vi "P3.6.vi"() -> ()   [LabVIEW 2020]
uses:
  <vilib>/Analysis/2dsp.llb/1D Convolution (DBL).vi
  <vilib>/Analysis/NI_AALPro.lvlib
panel:
  out "X * Y":dbl[](graph)
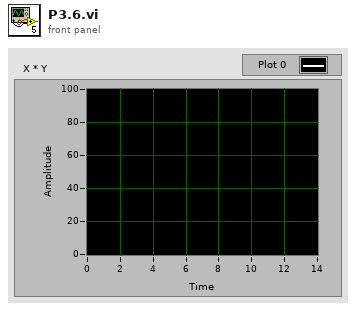
[diagram p1: front panel]
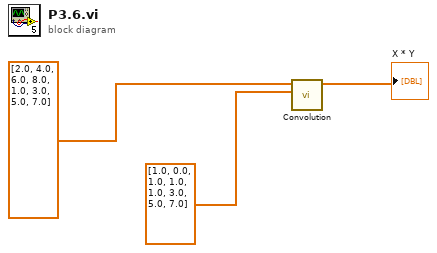
[diagram p0: block diagram]
diagram:
  n1 = call-poly <vilib>:"Convolution.vi"("Y"=dbl[] [1.0, 0.0, 1.0, 1.0, 1.0, 3.0, 5.0, 7.0], "X"=dbl[] [2.0, 4.0, 6.0, 8.0, 1.0, 3.0, 5.0, 7.0]) -> ("X * Y"=→"X * Y":dbl[])  [unwired: 8 in, 1 out]
